vi "check connect.vi"(8 "error in (no error)":errorcluster, 11 "VISA resource name":refnum<visa-resource-name>) -> (0 "error out":errorcluster, 2 "connectd":bool=TRUE, 3 "VISA resource name out":refnum<visa-resource-name>)   [LabVIEW 2016]
uses:
  global value.vi
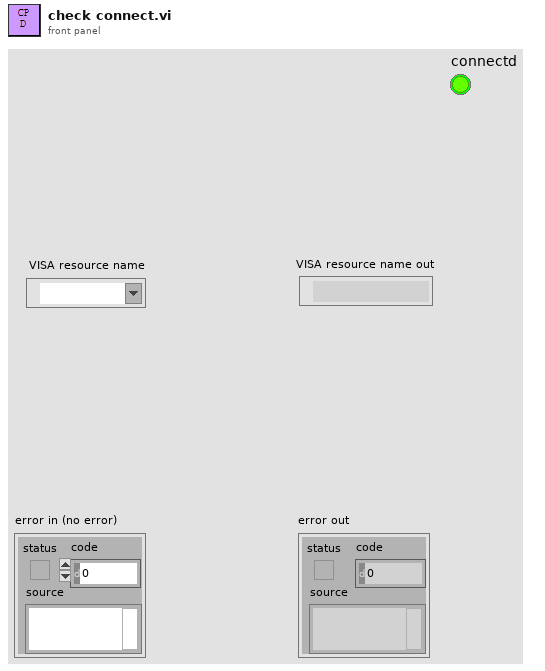
[diagram p1: front panel]
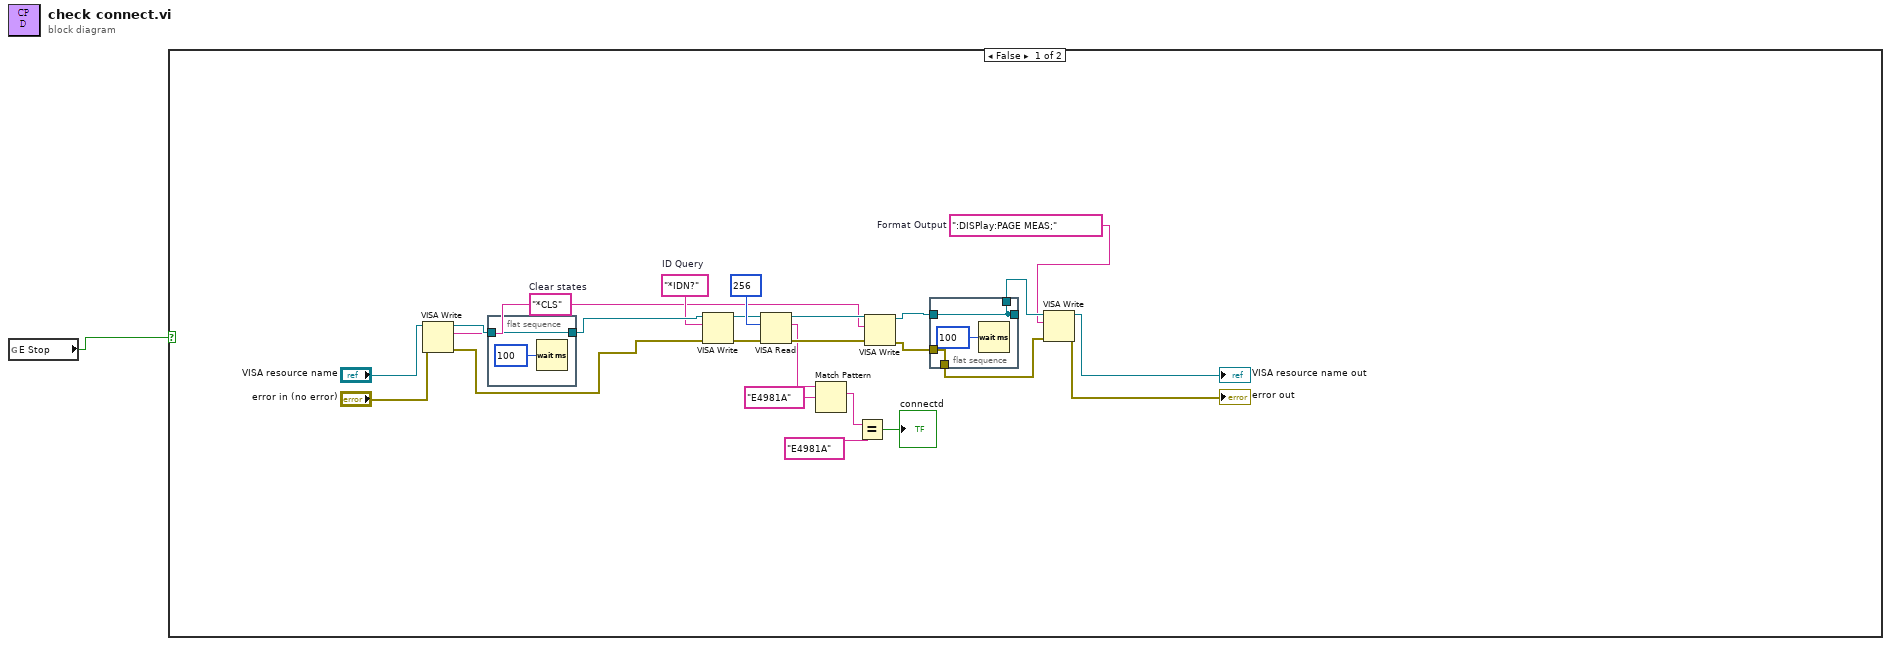
[diagram p0: block diagram]
diagram:
  n1 = global read "global value.vi" "E Stop"() -> (w1:bool)
  n2 = case shown="False" w1 {
    frame False {
      w21 = ":DISPlay:PAGE MEAS;"  # Format Output
      w2 = "*CLS"  # Clear states
      w13 = "*IDN?"  # ID Query
      n3 = VISA Write(VISA resource name="VISA resource name", write buffer=w2, error in (no error)="error in (no error)") -> (VISA resource name out=w18:refnum<visa-resource-name>, error out=w17:errorcluster)  [unwired: 1 out]
      n4 = flat-sequence {
        tunnel: [w29] -> w16
        tunnel: w18 -> [w29]
        frame #0 {
          n5 = Wait (ms)(milliseconds to wait=u32 100) -> ()  [unwired: 1 out]
        }
      }
      n6 = VISA Write(VISA resource name=w16, write buffer=w13, error in (no error)=w17) -> (VISA resource name out=w9:refnum<visa-resource-name>, error out=w10:errorcluster)  [unwired: 1 out]
      n7 = VISA Read(VISA resource name=w9, byte count=u32 256, error in (no error)=w10) -> (VISA resource name out=w19:refnum<visa-resource-name>, read buffer=w8:string, error out=w20:errorcluster)  [unwired: 1 out]
      n8 = Match Pattern(string=w8, regular expression="E4981A") -> (match substring=w14:string)  [unwired: 1 in, 3 out]
      n9 = Equal?(x=w14, y="E4981A") -> (x = y?=→"connectd":bool)
      n10 = VISA Write(VISA resource name=w19, write buffer=w2, error in (no error)=w20) -> (VISA resource name out=w22:refnum<visa-resource-name>, error out=w23:errorcluster)  [unwired: 1 out]
      n11 = flat-sequence {
        tunnel: [w26] -> _
        tunnel: w22 -> [w26]
        tunnel: w23 -> [w27]
        tunnel: [w27] -> w24
        tunnel: [w26] -> w25
        frame #0 {
          n12 = Wait (ms)(milliseconds to wait=u32 100) -> ()  [unwired: 1 out]
        }
      }
      n13 = VISA Write(VISA resource name=w25, write buffer=w21, error in (no error)=w24) -> (VISA resource name out=→"VISA resource name out":refnum<visa-resource-name>, error out=→"error out":errorcluster)  [unwired: 1 out]
    }
    frame True {
    }
  }
